vi "(SubVI) Calculate all frame BM.vi"(10 "y position (pixel)":dbl[](array[numeric]), 11 "x position (pixel)":dbl[](array[numeric])) -> (0 "y standard deviation":dbl, 3 "x standard deviation":dbl, 4 "y position (delete y fit error)":dbl[](array[numeric]), 5 "x position (delete x fit error)":dbl[](array[numeric]))   [LabVIEW 2016]
uses:
  <vilib>/Analysis/NI_AALBase.lvlib
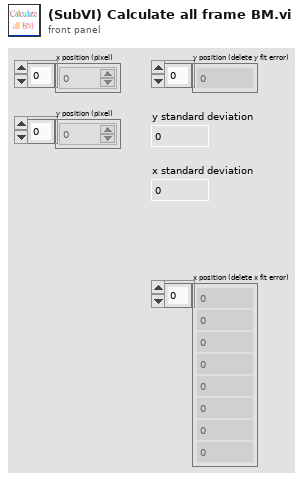
[diagram p1: front panel]
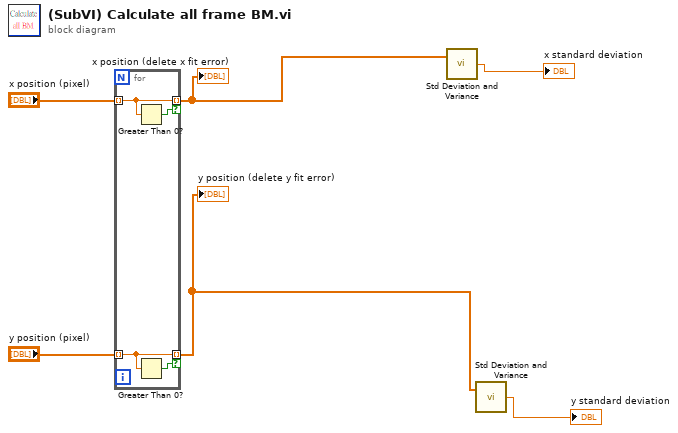
[diagram p0: block diagram]
diagram:
  n1 = for {
    tunnel: [w8] -> w2 mode=indexing if=w7
    tunnel: [w9] -> w4 mode=indexing if=w10
    tunnel: "x position (pixel)" -> [w9] mode=indexing
    tunnel: "y position (pixel)" -> [w8] mode=indexing
    n2 = Greater Than 0?(x=w9) -> (x > 0?=w10:bool)
    n3 = Greater Than 0?(x=w8) -> (x > 0?=w7:bool)
  }
  "y position (delete y fit error)" <- w2
  "x position (delete x fit error)" <- w4
  n4 = call <vilib>:"Std Deviation and Variance.vi"("X"=w4) -> ("standard deviation"=→"x standard deviation":dbl)  [unwired: 1 in, 2 out]
  n5 = call <vilib>:"Std Deviation and Variance.vi"("X"=w2) -> ("standard deviation"=→"y standard deviation":dbl)  [unwired: 1 in, 2 out]
